vi "CanChannelGetStatus.vi"(3 "error in":errorcluster {"code" format="%.0x"}, 5 "CAN Channel Handle in":u32 format="%x") -> (0 "error out":errorcluster {"code" format="%.0x"}, 1 "Channel Status":T1 {"TX Load (%)" max=100 scale=0.0..100.0; "RX Load (%)" max=100 scale=0.0..100.0; "Line Status"."BUS Timing"."BTR1" format="%02x"; "Line Status"."BUS Timing"."BTR0" format="%02x"; "Line Status"."BUS Load (%)" max=100 step=1 scale=0.0..100.0}, 2 "CAN Channel Handle out":u32)   [LabVIEW 2012]
doc: "Gets the status of the CAN channel."
uses:
  vcilva.dll
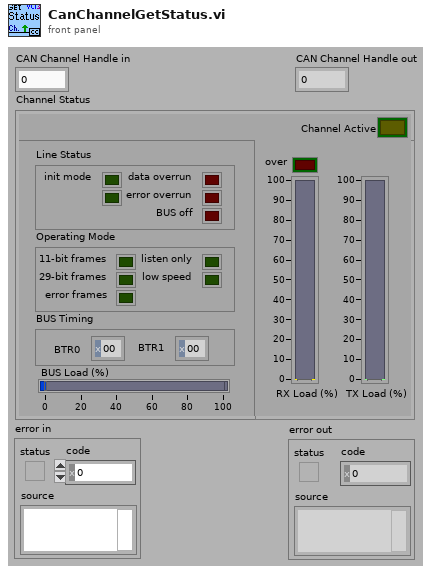
[diagram p1: front panel]
types:
  T1 = cluster{"Line Status":cluster{"Line Status":cluster{"init mode":bool, "TX pending":bool, "data overrun":bool, "error overrun":bool, "BUS off":bool}, "Operating Mode":cluster{"11-bit frames":bool, "29-bit frames":bool, "error frames":bool, "listen only":bool, "low speed":bool}, "BUS Timing":cluster{"BTR0":u8, "BTR1":u8}, "BUS Load (%)":u8}, "Channel Active":bool, "over":bool, "RX Load (%)":u8, "TX Load (%)":u8}
  T2 = cluster{"Line Status":cluster{"Line Status":cluster{"init mode":bool, "TX pending":bool, "data overrun":bool, "error overrun":bool, "BUS off":bool}, "Operating Mode":cluster{"11-bit frames":bool, "29-bit frames":bool, "error frames":bool, "listen only":bool, "low speed":bool}, "BUS Timing":cluster{"BTR0":u8, "BTR1":u8}, "BUS Load (%)":u8}, "Channel Active":bool, "RX FIFO overrun":bool, "RX FIFO Load (%)":u8, "TX FIFO Load (%)":u8}
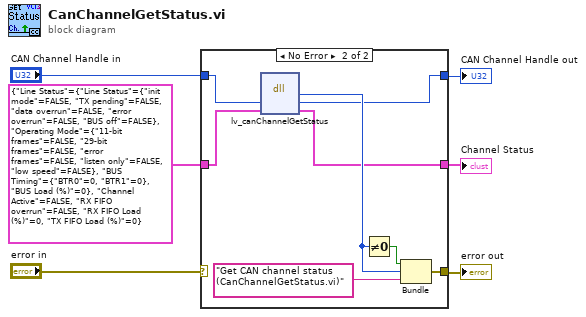
[diagram p0: block diagram]
diagram:
  n1 = case shown="No Error" "error in" {
    selector: "error in" -> [w9 _]
    tunnel: [w9 w17] -> w5
    tunnel: "CAN Channel Handle in" -> [w8 w13]
    tunnel: [w8 w12] -> w3
    tunnel: T2 {"Line Status"={"Line Status"={"init mode"=FALSE, "TX pending"=FALSE, "data overrun"=FALSE, "error overrun"=FALSE, "BUS off"=FALSE}, "Operating Mode"={"11-bit frames"=FALSE, "29-bit frames"=FALSE, "error frames"=FALSE, "listen only"=FALSE, "low speed"=FALSE}, "BUS Timing"={"BTR0"=0, "BTR1"=0}, "BUS Load (%)"=0}, "Channel Active"=FALSE, "RX FIFO overrun"=FALSE, "RX FIFO Load (%)"=0, "TX FIFO Load (%)"=0} ("Channel Status") -> [w7 w11]
    tunnel: [w7 w10] -> w1
    frame Error {
    }
    frame No Error {
      n2 = dll-call lib="vcilva.dll" fn="lv_canChannelGetStatus"("hCanChn"=w13, "Channel Status"=w11) -> (w14:i32, "hCanChn"=w12:u32, "Channel Status"=w10:T2)  [unwired: 3 in, 2 out]
      n3 = Not Equal To 0?(x=w14) -> (x != 0?=w16:bool)
      n4 = Bundle(w16, w14, "Get CAN channel status (CanChannelGetStatus.vi)") -> (w17:errorcluster)  [unwired: 1 in]
    }
  }
  "error out" <- w5
  "CAN Channel Handle out" <- w3
  "Channel Status" <- w1
